vi "ziExample-HF2-TipProtect.vi"() -> ()   [LabVIEW 2009]
doc: "Control a Zurich instrument device via the LabOne Labview API. \nRequirements: Zurich Instruments HF2.\nThis example controls the Tip Protect settings, which are not avialble in ziControl otherwise. This example is also availalbe in compiled form when ziControl is installed.\n\n© Zurich Instruments AG, www.zhinst.com"
uses:
  <instrlib>/Zurich Instruments LabOne/Public/Configure/ziSetValueDouble.vi
  <instrlib>/Zurich Instruments LabOne/Zurich Instruments LabOne.lvlib
panel:
  in  "stop":bool
  in  "Tab Control":enum32{"TipProtect"}(tab)
  out "pids/%u/tipprotect/active":bool caption="CF"
  out "wasectactive":bool caption="CF"
  in  "clearstatus":bool caption="defaultPhase"
  in  "pids/%u/tipprotect/activetimeconstant":dbl=1.0 caption="TC active (s)" format="%_4p"
  in  "pids/%u/tipprotect/inactivetimeconstant":dbl=0.001 caption="TC inactive (s)" format="%_4p"
  in  "tipprotect_auto_tc":bool caption="LI"
  in  "pids/%u/tipprotect/pll":i32(ring) caption="PLL" items=["1", "2"]
  in  "pids/%u/tipprotect/enable":bool caption="Tip Protect enable"
  in  "pid select":i32(ring) caption="PID" items=["1", "2", "3", "4"]
  out "PID active":bool caption="CF"
  in  "outputdefault":dbl=0.001 caption="Default output value" format="%_4p"
  # "TP active"
  # "PID enabled"
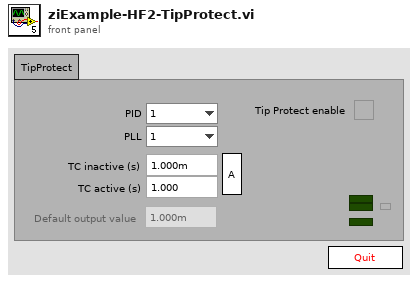
[diagram p1: front panel]
types:
  T1 = typedef "Zurich Instruments LabOne.lvlib/ziTypeHandle.ctl" = cluster{"handleValid":bool, "Conn":u64, "Path Prefix":string, "Handle":u64, "Connected":bool, "Clockbase(s)":dbl}
  T2 = enum32{"invalid app kind", "Development System", "Run Time System", "Student Edition", "Embedded LabVIEW", "Evaluation", "Custom"}
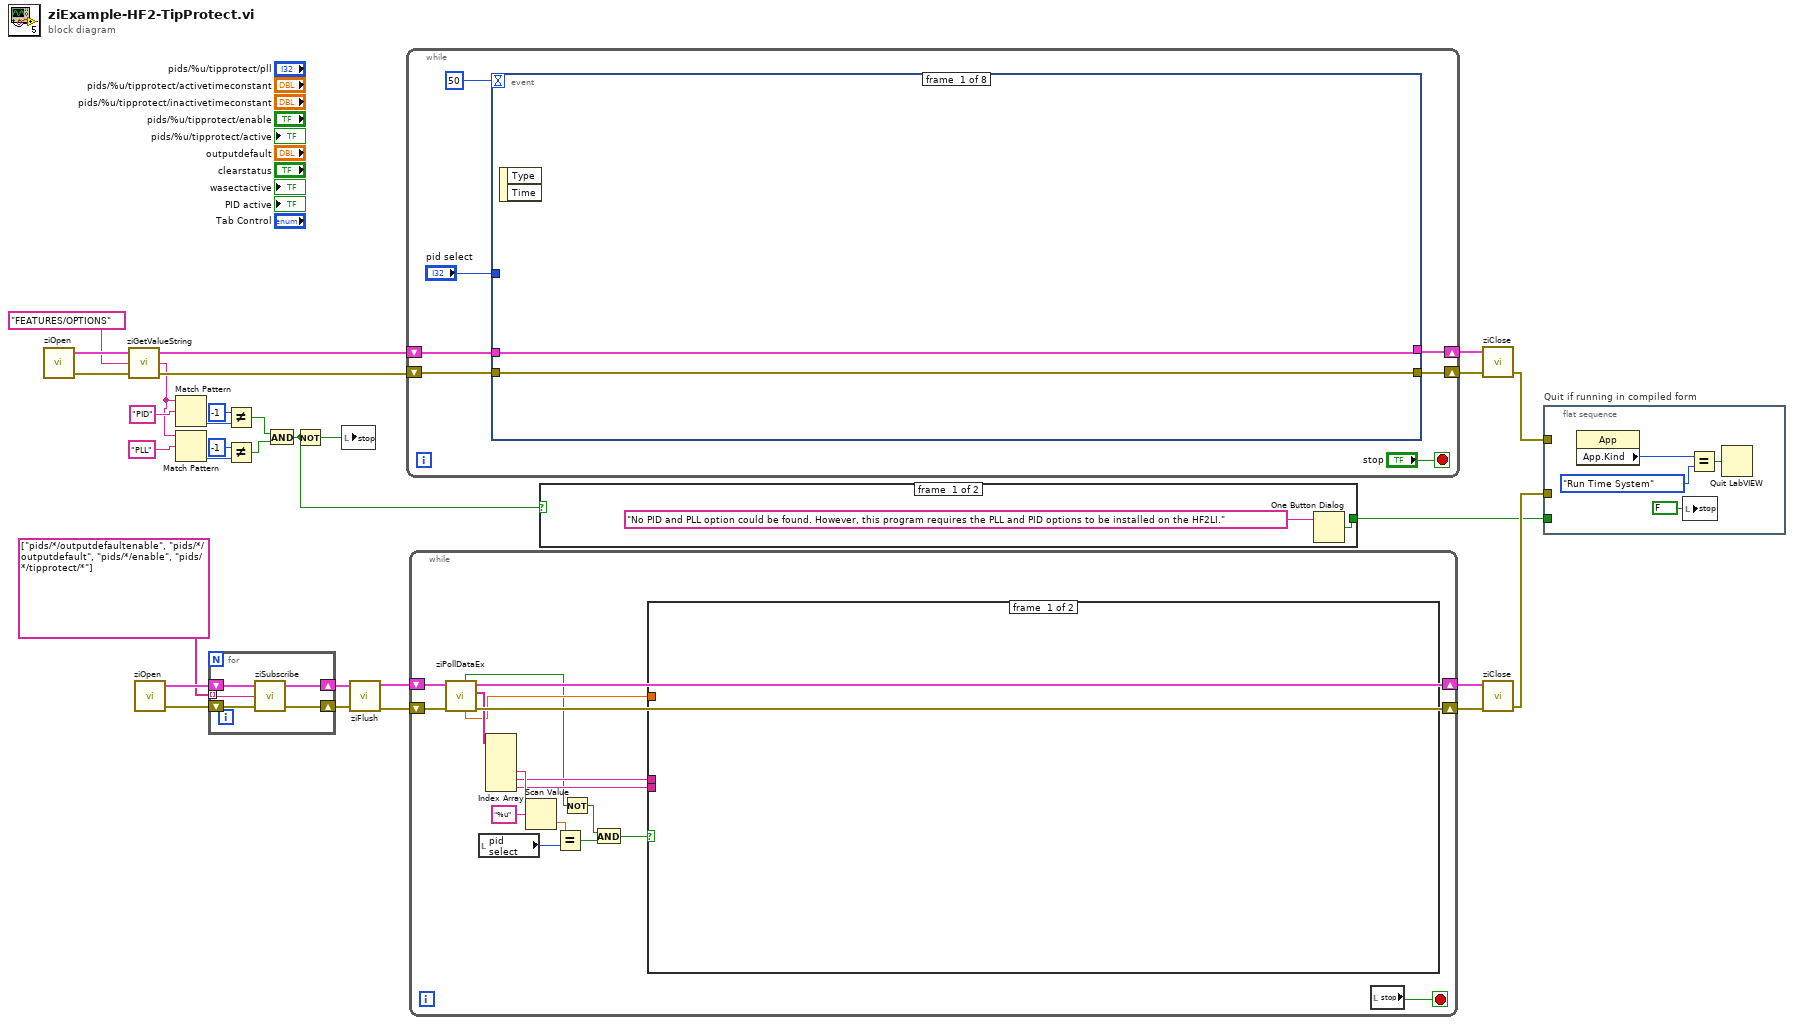
[diagram p0: block diagram]
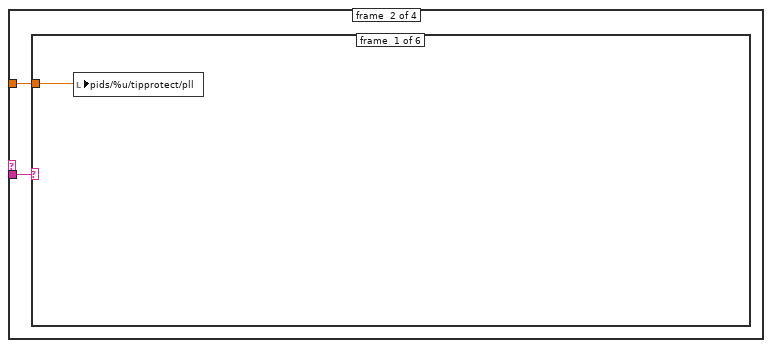
[diagram p4: hidden frame]
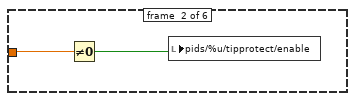
[diagram p5: hidden frame]
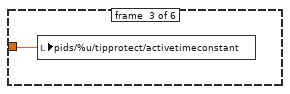
[diagram p6: hidden frame]
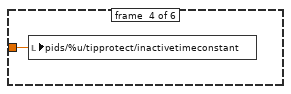
[diagram p7: hidden frame]
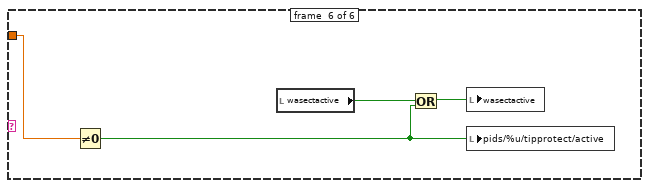
[diagram p9: hidden frame]
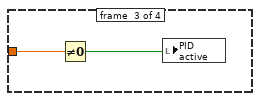
[diagram p10: hidden frame]
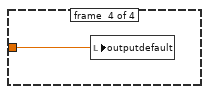
[diagram p11: hidden frame]
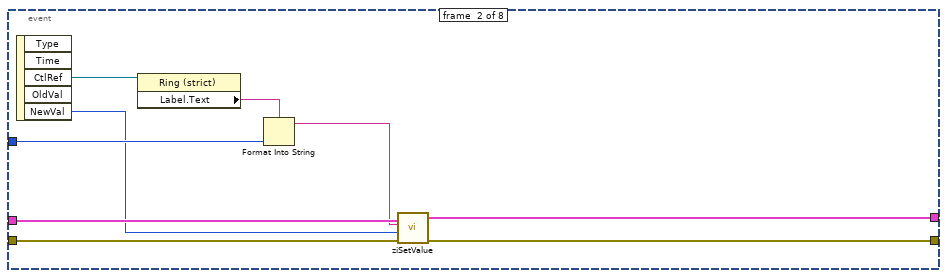
[diagram p12: hidden frame]
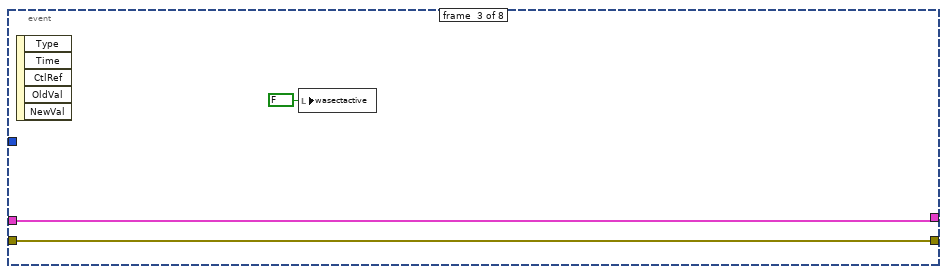
[diagram p13: hidden frame]
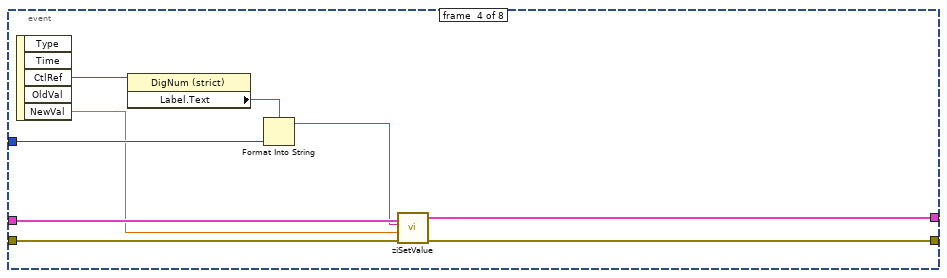
[diagram p14: hidden frame]
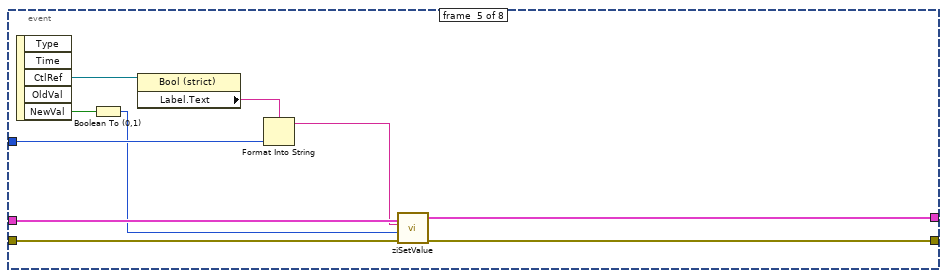
[diagram p15: hidden frame]
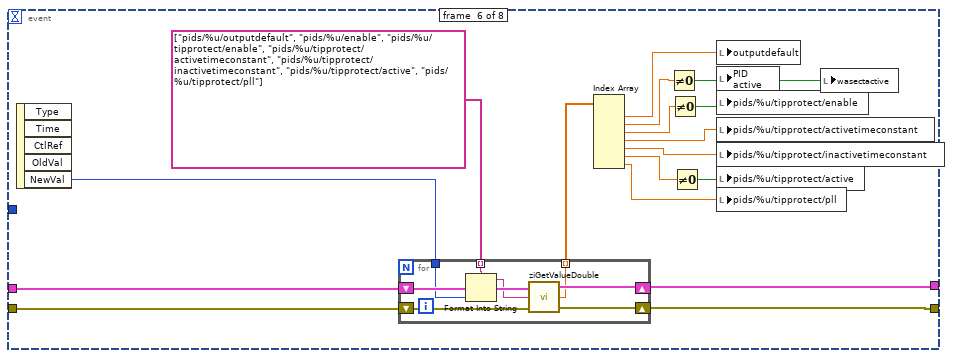
[diagram p16: hidden frame]
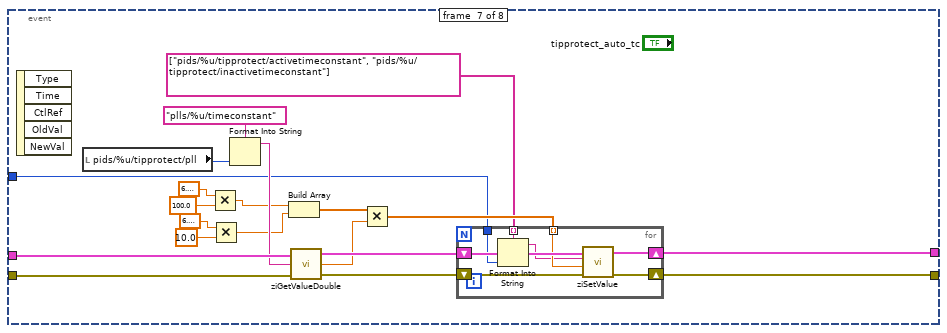
[diagram p17: hidden frame]
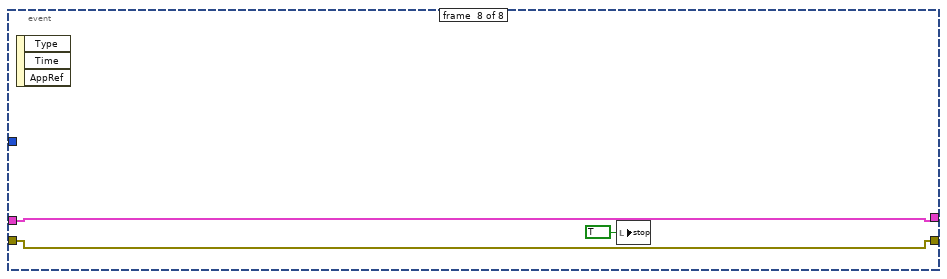
[diagram p18: hidden frame]
diagram:
  n1 = call <instrlib>:"ziOpen.vi"() -> ("Error Out"=w17:errorcluster, "HandleOut"=w16:T1)  [unwired: 4 in, 1 out]
  n2 = call <instrlib>:"ziGetValueString.vi"("error in"=w17, "Path"="FEATURES/OPTIONS", "Handle In"=w16) -> ("error out"=w14:errorcluster, "Value"=w4:string, "Handle Out"=w15:T1)
  n3 = call <instrlib>:"ziOpen.vi"() -> ("Error Out"=w29:errorcluster, "HandleOut"=w30:T1)  [unwired: 4 in, 1 out]
  n4 = Match Pattern(string=w4, regular expression="PID") -> (offset past match=w10:i32)  [unwired: 4 out]
  n5 = Match Pattern(string=w4, regular expression="PLL") -> (offset past match=w9:i32)  [unwired: 4 out]
  n6 = for {
    tunnel: string[] ["pids/*/outputdefaultenable", "pids/*/outputdefault", "pids/*/enable", "pids/*/tipprotect/*"] -> [w31] mode=indexing
    shift-right: [w33] -> w28
    shift-left: w30 -> [w35]
    shift-right: [w32] -> w27
    shift-left: w29 -> [w34]
    n7 = call <instrlib>:"ziSubscribe.vi"("error in"=w34, "Path ()"=w31, "Handle In"=w35) -> ("error out"=w32:errorcluster, "Handle Out"=w33:T1)  [unwired: 1 in]
  }
  n8 = Not Equal?(x=-1, y=w10) -> (x != y?=w5:bool)
  n9 = Not Equal?(x=-1, y=w9) -> (x != y?=w6:bool)
  n10 = And(x=w5, y=w6) -> (x .and. y?=w2:bool)
  n11 = Not(x=w2) -> (.not. x?=w3:bool)
  n12 = local write "stop"(w3) -> ()
  n13 = call <instrlib>:"ziFlush.vi"("error in"=w27, "Handle In"=w28) -> ("error out"=w25:errorcluster, "Handle Out"=w26:T1)  [unwired: 8 in]
  n14 = while {
    shift-right: [w40] -> w22
    shift-left: w15 -> [w41]
    shift-right: [w39] -> w21
    shift-left: w14 -> [w38]
    stop <- "stop" stop-if-true
    n15 = event shown="[7] Application Instance Close" {
      selector: _ -> [_ _ _ _ _ _ _ _]
      dyn-events: _ -> [_ _ _ _ _ _ _ _]
      timeout: 50 ("TimeOut ms (50)") -> [_ _ _ _ _ _ _ _]
      tunnel: "pid select" -> [_ w51 _ w62 w71 _ w106 _]
      tunnel: w41 -> [w44 w50 w54 w61 w70 w89 w117 w127]
      tunnel: [w44 w49 w54 w60 w69 w88 w113 w127] -> w40
      tunnel: [w43 w48 w53 w59 w68 w86 w112 w126] -> w39
      tunnel: w38 -> [w43 w48 w53 w59 w68 w87 w116 w126]
      event #0 {
        n16 = event-data() -> ()  [unwired: 1 in, 2 out]
      }
      event #1 {
        n17 = event-data() -> ("CtlRef"=w52:refnum<vi>, "NewVal"=w46:i32)  [unwired: 1 in, 3 out]
        n18 = property class="Ring (strict)"(reference=w52) -> ("Label.Text"=w45:string)  [unwired: 1 in, 2 out]
        n19 = Format Into String(format string=w45, w51) -> (resulting string=w47:string)  [unwired: 2 in, 1 out]
        n20 = call-poly <instrlib>:"ziSetValue.vi"("Value"=w46, "Path"=w47, "Handle In"=w50) -> ("Handle Out"=w49:T1)  [unwired: 2 in, 1 out]
      }
      event #2 {
        n21 = event-data() -> ()  [unwired: 1 in, 5 out]
        n22 = local write "wasectactive"(FALSE ("wasectactive")) -> ()
      }
      event #3 {
        n23 = event-data() -> ("CtlRef"=w63:refnum<vi>, "NewVal"=w57:dbl)  [unwired: 1 in, 3 out]
        n24 = property class="DigNum (strict)"(reference=w63) -> ("Label.Text"=w56:string)  [unwired: 1 in, 2 out]
        n25 = Format Into String(format string=w56, w62) -> (resulting string=w58:string)  [unwired: 2 in, 1 out]
        n26 = call-poly <instrlib>:"ziSetValue.vi"("Value"=w57, "Path"=w58, "Handle In"=w61) -> ("Handle Out"=w60:T1)  [unwired: 2 in, 1 out]
      }
      event #4 {
        n27 = event-data() -> ("CtlRef"=w72:refnum<vi>, "NewVal"=w66:bool)  [unwired: 1 in, 3 out]
        n28 = Boolean To (0,1)(Boolean=w66) -> (0, 1=w65:i16)
        n29 = property class="Bool (strict)"(reference=w72) -> ("Label.Text"=w64:string)  [unwired: 1 in, 2 out]
        n30 = Format Into String(format string=w64, w71) -> (resulting string=w67:string)  [unwired: 2 in, 1 out]
        n31 = call-poly <instrlib>:"ziSetValue.vi"("Value"=w65, "Path"=w67, "Handle In"=w70) -> ("Handle Out"=w69:T1)  [unwired: 2 in, 1 out]
      }
      event #5 {
        n32 = event-data() -> ("NewVal"=w74:i32)  [unwired: 1 in, 4 out]
        n33 = for {
          shift-right: [w96] -> w88
          shift-left: w89 -> [w97]
          shift-right: [w94] -> w86
          shift-left: w87 -> [w95]
          tunnel: string[] ["pids/%u/outputdefault", "pids/%u/enable", "pids/%u/tipprotect/enable", "pids/%u/tipprotect/activetimeconstant", "pids/%u/tipprotect/inactivetimeconstant", "pids/%u/tipprotect/active", "pids/%u/tipprotect/pll"] -> [w91] mode=indexing
          tunnel: [w93] -> w84 mode=indexing
          tunnel: w74 -> [w90]
          n34 = Format Into String(format string=w91, w90) -> (resulting string=w92:string)  [unwired: 2 in, 1 out]
          n35 = call <instrlib>:"ziGetValueDouble.vi"("error in"=w95, "Path"=w92, "Handle in"=w97) -> ("error out"=w94:errorcluster, "Value"=w93:dbl, "Handle out"=w96:T1)
        }
        n36 = Index Array(array=w84) -> (element #1=w83:dbl, element #2=w82:dbl, element #3=w80:dbl, element #4=w79:dbl, element #5=w78:dbl, element #6=w76:dbl, element #7=w75:dbl)  [unwired: 7 in]
        n37 = Not Equal To 0?(x=w82) -> (x != 0?=w73:bool)
        n38 = Not Equal To 0?(x=w80) -> (x != 0?=w81:bool)
        n39 = Not Equal To 0?(x=w76) -> (x != 0?=w77:bool)
        n40 = local write "outputdefault"(w83) -> ()
        n41 = local write "PID active"(w73) -> ()
        n42 = local write "pids/%u/tipprotect/enable"(w81) -> ()
        n43 = local write "pids/%u/tipprotect/activetimeconstant"(w79) -> ()
        n44 = local write "pids/%u/tipprotect/inactivetimeconstant"(w78) -> ()
        n45 = local write "pids/%u/tipprotect/active"(w77) -> ()
        n46 = local write "pids/%u/tipprotect/pll"(w75) -> ()
        n47 = local write "wasectactive"(w73) -> ()
      }
      event #6 {
        n48 = event-data() -> ()  [unwired: 1 in, 5 out]
        n49 = local read "pids/%u/tipprotect/pll"() -> (w105:i32)
        n50 = Multiply(x=6.283185307179586, y=100.0 ("x")) -> (x*y=w100:dbl)
        n51 = Multiply(x=6.283185307179586, y=10.0 ("x")) -> (x*y=w99:dbl)
        n52 = Format Into String(format string="plls/%u/timeconstant" ("path"), w105) -> (resulting string=w110:string)  [unwired: 2 in, 1 out]
        n53 = Build Array(w100, w99) -> (w98:dbl[])
        n54 = call <instrlib>:"ziGetValueDouble.vi"("error in"=w116, "Path"=w110, "Handle in"=w117) -> ("error out"=w114:errorcluster, "Value"=w109:dbl, "Handle out"=w115:T1)
        n55 = Multiply(x=w98, y=w109) -> (x*y=w108:dbl[])
        n56 = for {
          tunnel: w108 -> [w121] mode=indexing
          tunnel: string[] ["pids/%u/tipprotect/activetimeconstant", "pids/%u/tipprotect/inactivetimeconstant"] -> [w120] mode=indexing
          shift-right: [w123] -> w113
          shift-left: w115 -> [w125]
          shift-right: [w122] -> w112
          shift-left: w114 -> [w124]
          tunnel: w106 -> [w119]
          n57 = Format Into String(format string=w120, w119) -> (resulting string=w118:string)  [unwired: 2 in, 1 out]
          n58 = call-poly <instrlib>:"ziSetValue.vi"("Error In"=w124, "Value"=w121, "Path"=w118, "Handle In"=w125) -> ("Error Out"=w122:errorcluster, "Handle Out"=w123:T1)  [unwired: 1 in]
        }
      }
      event #7 {
        n59 = event-data() -> ()  [unwired: 1 in, 3 out]
        n60 = local write "stop"(TRUE ("stop")) -> ()
      }
    }
  }
  n61 = while {
    shift-right: [w143] -> w24
    shift-left: w26 -> [w145]
    shift-right: [w142] -> w23
    shift-left: w25 -> [w144]
    stop <- w140 stop-if-true
    n62 = call <instrlib>:"ziPollDataEx.vi"("error in"=w144, "Handle In"=w145) -> ("error out"=w142:errorcluster, "PathArray"=w141:string[], "Handle Out"=w143:T1, "Value Double"=w132:dbl, "Timed Out"=w130:bool)  [unwired: 2 in, 3 out]
    n63 = local read "pid select"() -> (w139:i32)
    n64 = Index Array(array=w141) -> (element #3=w136:string, element #4=w134:string, element #5=w135:string)  [unwired: 5 in, 2 out]
    n65 = Scan Value(string=w136, format string="%u") -> (value=w138:dbl)  [unwired: 1 in, 1 out]
    n66 = Equal?(x=w138, y=w139) -> (x = y?=w133:bool)
    n67 = Not(x=w130) -> (.not. x?=w129:bool)
    n68 = And(x=w129, y=w133) -> (x .and. y?=w131:bool)
    n69 = case shown="True" w131 {
      tunnel: w135 -> [_ w148]
      tunnel: w132 -> [_ w147]
      tunnel: w134 -> [_ w146]
      frame #0 {
      }
      frame #1 {
        n70 = case shown="\"TIPPROTECT\"" w146 {
          tunnel: w148 -> [_ w150 _ _]
          tunnel: w147 -> [_ w149 w161 w162]
          frame #0 {
          }
          frame #1 {
            n71 = case shown="\"INACTIVETIMECONSTANT\"" w150 {
              tunnel: w149 -> [w151 w153 w154 w155 _ w156]
              frame #0 {
                n72 = local write "pids/%u/tipprotect/pll"(w151) -> ()
              }
              frame #1 {
                n73 = Not Equal To 0?(x=w153) -> (x != 0?=w152:bool)
                n74 = local write "pids/%u/tipprotect/enable"(w152) -> ()
              }
              frame #2 {
                n75 = local write "pids/%u/tipprotect/activetimeconstant"(w154) -> ()
              }
              frame #3 {
                n76 = local write "pids/%u/tipprotect/inactivetimeconstant"(w155) -> ()
              }
              frame #4 {
              }
              frame #5 {
                n77 = Not Equal To 0?(x=w156) -> (x != 0?=w157:bool)
                n78 = local read "wasectactive"() -> (w159:bool)
                n79 = Or(x=w159, y=w157) -> (x .or. y?=w158:bool)
                n80 = local write "wasectactive"(w158) -> ()
                n81 = local write "pids/%u/tipprotect/active"(w157) -> ()
              }
            }
          }
          frame #2 {
            n82 = Not Equal To 0?(x=w161) -> (x != 0?=w160:bool)
            n83 = local write "PID active"(w160) -> ()
          }
          frame #3 {
            n84 = local write "outputdefault"(w162) -> ()
          }
        }
      }
    }
    n85 = local read "stop"() -> (w140:bool)
  }
  n86 = case shown="False" w2 {
    tunnel: [w163 _] -> w1
    frame #0 {
      n87 = One Button Dialog(message="No PID and PLL option could be found. However, this program requires the PLL and PID options to be installed on the HF2LI.") -> (true=w163:bool)  [unwired: 1 in]
    }
    frame #1 {
    }
  }
  n88 = call <instrlib>:"ziClose.vi"("Error In"=w21, "Handle In"=w22) -> ("Error Out"=w19:errorcluster)  [unwired: 2 in, 1 out]
  n89 = call <instrlib>:"ziClose.vi"("Error In"=w23, "Handle In"=w24) -> ("Error Out"=w18:errorcluster)  [unwired: 2 in, 1 out]
  n90 = flat-sequence "Quit if running in compiled form" {
    tunnel: w19 -> [_]
    tunnel: w18 -> [_]
    tunnel: w1 -> [_]
    frame #0 {
      n91 = property class="App"() -> ("App.Kind"=w168:T2)  [unwired: 2 in, 2 out]
      n92 = local write "stop"(FALSE ("stop")) -> ()
      n93 = Equal?(x=w168, y=T2."Run Time System" ("Application:Kind")) -> (x = y?=w166:bool)
      n94 = Quit LabVIEW(quit? (T)=w166) -> ()
    }
  }
